vi "Longer Pump dLSP501 Read System Status.vi"() -> ()   [LabVIEW 2023, in "Longer Pump dLSP501 Series.lvlib"]
uses:
  <instrlib>/Longer Pump dLSP501 Modbus RTU Series/Longer Pump dLSP501 Series.lvlib
  <instrlib>/Longer Pump dLSP501 Modbus RTU Series/Private/Initialize - Integrated Address.vi
  <vilib>/NI/Modbus Library/API/Master/Modbus Master.lvclass
  <vilib>/NI/Modbus Library/API/Modbus API.lvclass
  C:/Program Files/National Instruments/LabVIEW 2023/vi.lib/NI/Modbus Library/API/Modbus API.lvclass
panel:
  out "Error out":errorcluster caption="错误输出"
  in  "Error in":errorcluster caption="错误输入"
  in  "Open Port":bool caption="打开串口"
  out "Run Information":string caption="运行信息"
  out "Error Information":string caption="错误信息"
  in  "Close Port":bool caption="关闭串口"
  in  "Communication Config":T1={"Address"=1, "Baud Rate"=115200, "Parity"=0} caption="通讯设置" {"Parity" items=["无校验", "奇校验", "偶校验", "标记", "空格"]; "Baud Rate" items=["1200"=1200, "2400"=2400, "9600"=9600, "19200"=19200, "38400"=38400, "57600"=57600, "115200"=115200]}
  in  "VISA resource name":refnum<visa-resource-name>="COM1" caption="VISA资源名"
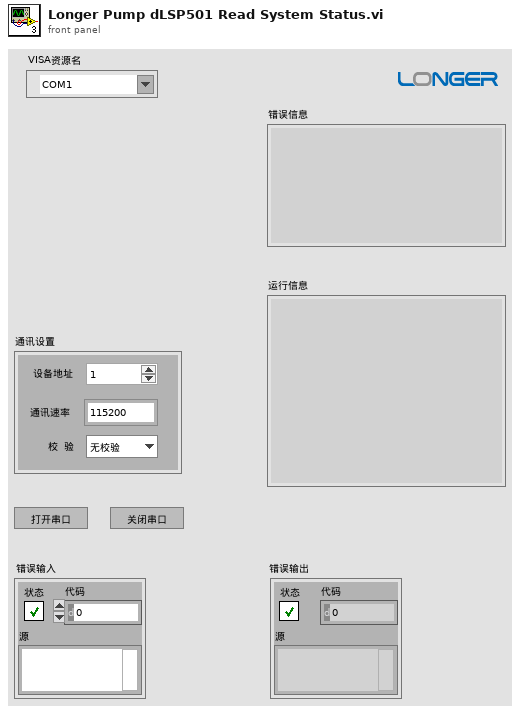
[diagram p1: front panel]
types:
  T1 = cluster{"Address":u8, "Baud Rate":u32, "Parity":u16}
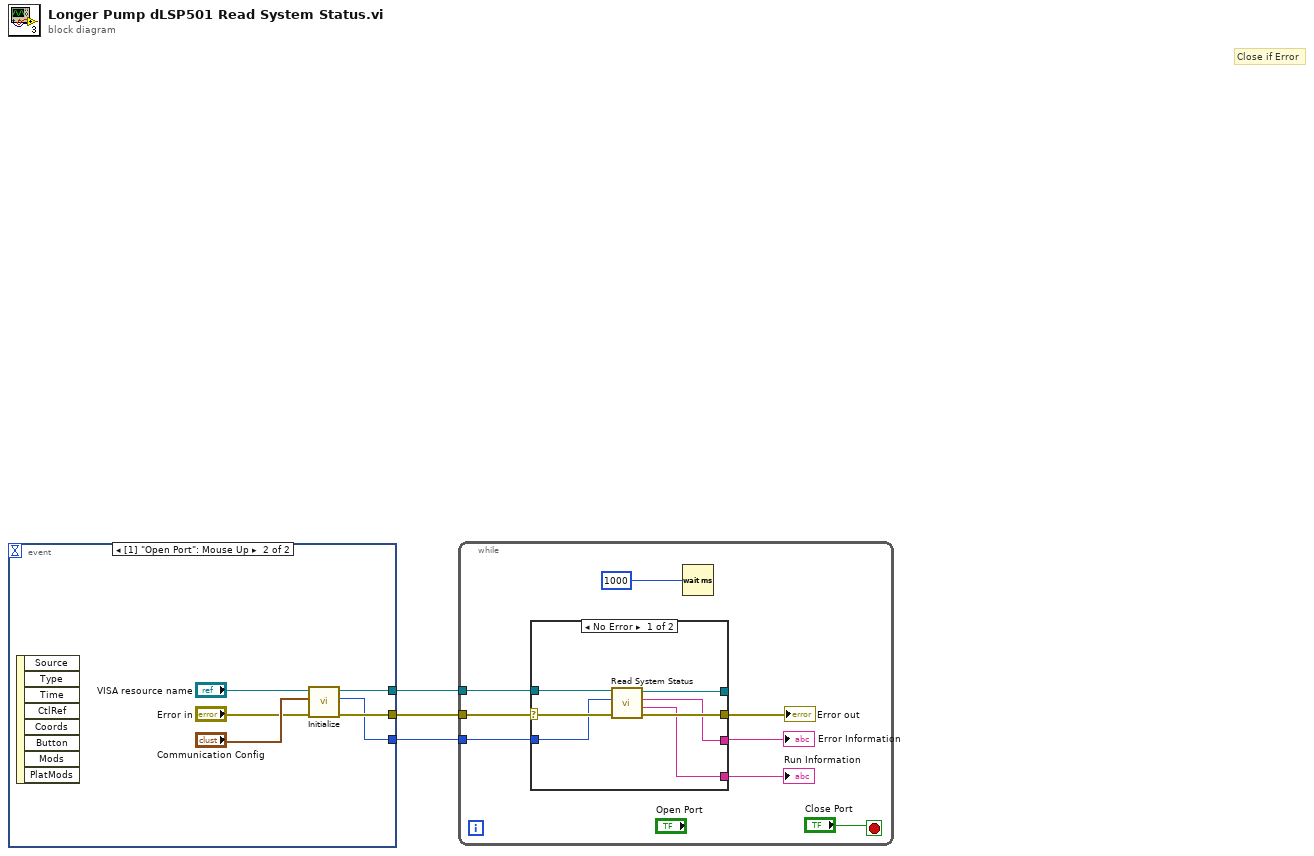
[diagram p0: block diagram]
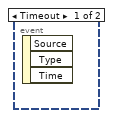
[diagram p2: hidden frame]
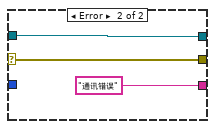
[diagram p3: hidden frame]
diagram:
  # "Close if Error"
  n1 = event shown="[1] \"Open Port\": Mouse Up" {
    selector: _ -> [_ _]
    dyn-events: _ -> [_ _]
    timeout: _ -> [_ _]
    tunnel: [_ w7] -> w3
    tunnel: [_ w6] -> w2
    tunnel: [_ w5] -> w1
    event Timeout {
      n2 = event-data() -> ()  [unwired: 1 in, 3 out]
    }
    event "Open Port": Mouse Up {
      n3 = event-data() -> ()  [unwired: 1 in, 8 out]
      n4 = call-poly <instrlib>:"Initialize.vi"("Error in"="Error in", "Comm. Config"="Communication Config", "VISA resource name"="VISA resource name") -> ("Error out"=w7:errorcluster, "Channel"=w6:i32, "serial master instance"=w5:refnum<class "Modbus Master.lvclass">)  [unwired: 5 in]
    }
  }
  n5 = while {
    tunnel: w3 -> [w17]
    tunnel: w1 -> [w16]
    tunnel: w2 -> [w12]
    stop <- "Close Port" stop-if-true
    n6 = case shown="No Error" w17 {
      selector: w17 -> [w23 w26]
      tunnel: w16 -> [w24 w27]
      tunnel: [w21 w27] -> _
      tunnel: [w22 w26] -> w10
      tunnel: [w18 _] -> w11
      tunnel: [w19 "通讯错误"] -> w13
      tunnel: w12 -> [w20 _]
      frame No Error {
        n7 = call <instrlib>:"Read System Status.vi"("Error in"=w23, "Channel"=w20, "Modbus master in"=w24) -> ("Error out"=w22:errorcluster, "Run Status Information"=w18:string, "Error Information"=w19:string, "Modbus instance out"=w21:refnum<class "Modbus API.lvclass">)  [unwired: 5 in]
      }
      frame Error {
      }
    }
    "Error Information" <- w13
    "Run Information" <- w11
    "Error out" <- w10
    n8 = Wait (ms)(milliseconds to wait=u32 1000 ("等待时间（毫秒）")) -> ()  [unwired: 1 out]
  }
